vi "find_max_min.vi"(7 "FWHM(T)?":bool, 9 "w Array":dbl[](array[numeric]) format="%.2f", 10 "z Array":dbl[](array[numeric]) format="%.2f") -> (0 "FWHM":dbl format="%.5f", 1 "min w":dbl format="%.5f", 2 "min  z":dbl format="%.2f", 3 "contains waist?":bool)   [LabVIEW 2016]
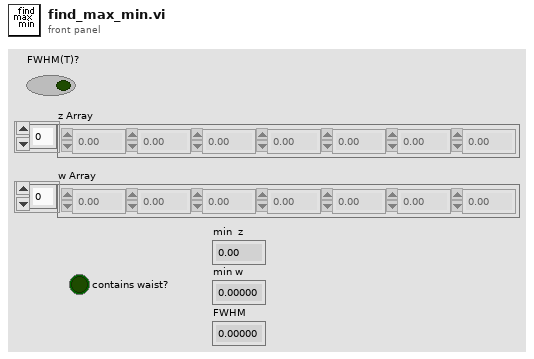
[diagram p1: front panel]
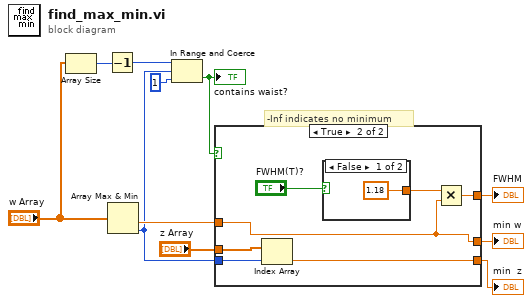
[diagram p0: block diagram]
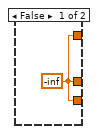
[diagram p2: hidden frame]
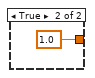
[diagram p3: hidden frame]
diagram:
  # "-Inf indicates no minimum"
  n1 = Array Size(array="w Array") -> (size(s)=w6:i32)
  n2 = Decrement(x=w6) -> (x-1=w4:i32)
  n3 = Array Max & Min(array="w Array") -> (min value=w11:dbl, min index (indices)=w10:i32)  [unwired: 2 out]
  n4 = In Range and Coerce(upper limit=w4, x=w10, lower limit=1) -> (In Range?=w2:bool)  [unwired: 1 out]
  "contains waist?" <- w2
  n5 = case shown="True" w2 {
    tunnel: w11 -> [_ w13]
    tunnel: w10 -> [_ w19]
    tunnel: [w12 w18] -> w9
    tunnel: [w12 w17] -> w8
    tunnel: "z Array" -> [_ w16]
    tunnel: [w12 w13] -> w1
    frame False {
      w12 = -inf
    }
    frame True {
      n6 = Index Array(array=w16, index=w19) -> (element=w18:dbl)
      n7 = case shown="False" "FWHM(T)?" {
        tunnel: [1.18 ("x") 1.0 ("x")] -> w15
        frame False {
        }
        frame True {
        }
      }
      n8 = Multiply(x=w15, y=w13) -> (x*y=w17:dbl)
    }
  }
  "min w" <- w1
  "min  z" <- w9
  "FWHM" <- w8
